vi "Centroid Calc.vi"(10 "Array":T1[](array[typedef])) -> (1 "Y Centroid":dbl, 2 "X Centroid":dbl)   [LabVIEW 2017]
uses:
  040-typeDefs/LidarPoint.ctl
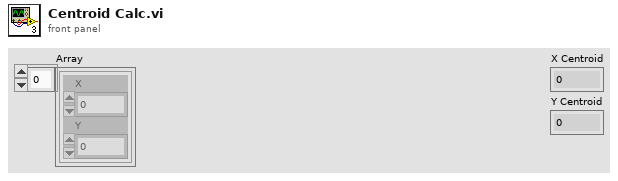
[diagram p1: front panel]
types:
  T1 = typedef "LidarPoint.ctl" = cluster{"X":dbl, "Y":dbl}
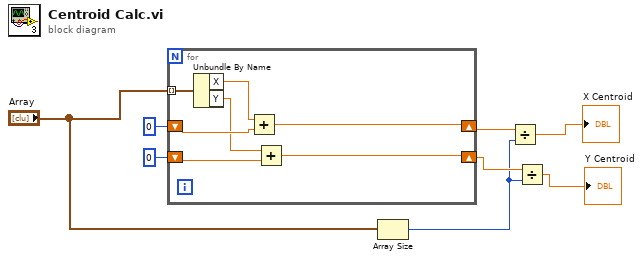
[diagram p0: block diagram]
diagram:
  n1 = for {
    tunnel: "Array" -> [w15] mode=indexing
    shift-right: [w10] -> w5
    shift-left: 0 -> [w14]
    shift-right: [w9] -> w4
    shift-left: 0 -> [w13]
    n2 = Unbundle By Name(w15) -> ("X"=w11:dbl, "Y"=w12:dbl)
    n3 = Add(x=w11, y=w14) -> (x+y=w10:dbl)
    n4 = Add(x=w12, y=w13) -> (x+y=w9:dbl)
  }
  n5 = Array Size(array="Array") -> (size(s)=w3:i32)
  n6 = Divide(x=w5, y=w3) -> (x/y=→"X Centroid":dbl)
  n7 = Divide(x=w4, y=w3) -> (x/y=→"Y Centroid":dbl)
